vi "InitialSMT1.vi"(8 "error in (no error)":errorcluster, 11 "Programing Logic in":refnum<class "Programing Logic.lvclass">) -> (0 "error out":errorcluster, 3 "Programing Logic out":refnum<class "Programing Logic.lvclass">)   [LabVIEW 2014, in "Programing Logic.lvclass"]
uses:
  Programing Logic.lvclass
  Programing Logic.lvclass/Programing Logic.ctl
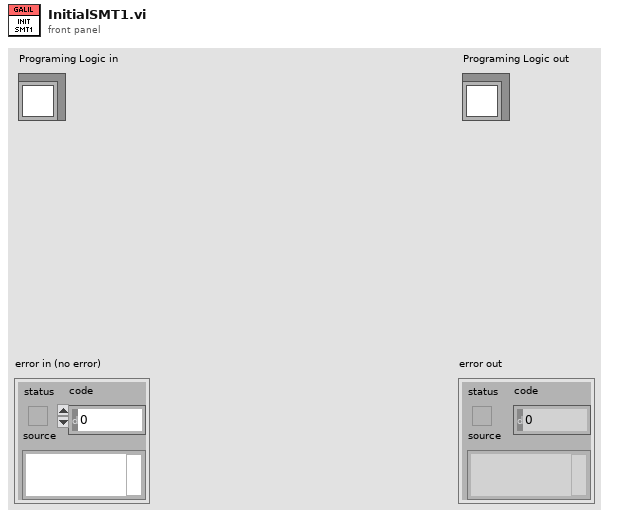
[diagram p1: front panel]
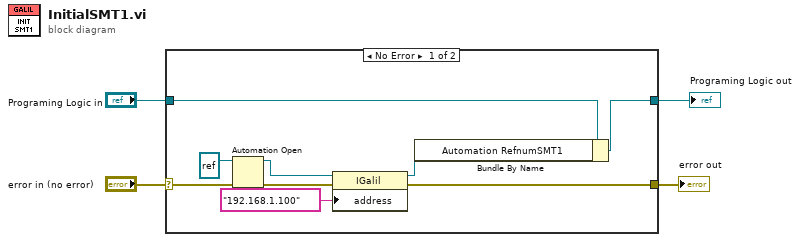
[diagram p0: block diagram]
diagram:
  n1 = case shown="No Error" "error in (no error)" {
    selector: "error in (no error)" -> [w12 w15]
    tunnel: [w8 w15] -> w3
    tunnel: [w6 w14] -> w1
    tunnel: "Programing Logic in" -> [w7 w14]
    frame No Error {
      n2 = Automation Open(error in (no error)=w12, Automation Refnum=refnum<k7> refnum ("Automation Refnum in")) -> (Automation Refnum=w11:refnum<k7>, error out=w10:errorcluster)  [unwired: 2 in]
      n3 = property on="Property Node" class="IGalil"(reference=w11, error in=w10, "address"="192.168.1.100") -> (reference out=w5:refnum<k7>, error out=w8:errorcluster)
      n4 = Bundle By Name(cluster=w7, "Automation RefnumSMT1"=w5) -> (w6:refnum<class "Programing Logic.lvclass">)
    }
    frame Error {
    }
  }
  "error out" <- w3
  "Programing Logic out" <- w1
